vi "LauncherFeeder.vi"(3 "Target RPM F":dbl=770.0, 4 "Target RPM":dbl=3300.0) -> (0 "RPM F":dbl=3319.8279051826034, 1 "RPM L":dbl=3319.8279051826034)   [LabVIEW 2016]
doc: "This example shows how to move a motor connected to an encoder and a wheel, and then read information about the system from an encoder.\n\nThis is an example of how to use feedback (from the encoder) to create an open loop system. If some control method was used, for example using PID, a closed loop system could be created.\n\nThis example expects a USB cable connected from your development PC to the Type B USB Jack (next to the power input) on the roboRIO.\n\nThis example requires the Driver Station to be running with Teleoperated Enabled."
uses:
  <vilib>/Rock Robotics/WPI/Utilities/WPI_GetSetVariantRefNum.vi
  <vilib>/gmath/NI_Gmath.lvlib
panel:
  in  "Feeder Enabled":bool=TRUE
  out "DS Original F":dbl=0.6428571428571428
  in  "Lower Limit F":dbl=-50.0 format="%#_13g"
  in  "Upper Limit F":dbl=50.0 format="%#_13g"
  in  "Pos Drive Signal F":dbl=0.4
  in  "Neg Drive Signal F":dbl=0.05
  out "Error F":dbl=-19.827905182603445
  out "Encoder Alarm Status F":string="Encoder Moving"
  out "Encoder Direction F":string="Forward"
  in  "Lower Limit L":dbl=-50.0 format="%#_13g"
  in  "Upper Limit L":dbl=50.0 format="%#_13g"
  out "Error L":dbl=-19.827905182603445
  out "DS Original L":dbl=0.6428571428571428
  in  "Neg Drive Signal":dbl=0.6
  in  "Pos Drive Signal":dbl=1.0
  in  "MS to Wait":u32=10
  out "Loop Time (s)":dbl=0.010378 format="%_6f"
  out "Encoder Alarm Status L":string="Encoder Moving"
  out "Encoder Direction L":string="Forward"
  # "These can be set while running."
  # "Output information."
  # "Need to tune target RPM and drive signals"
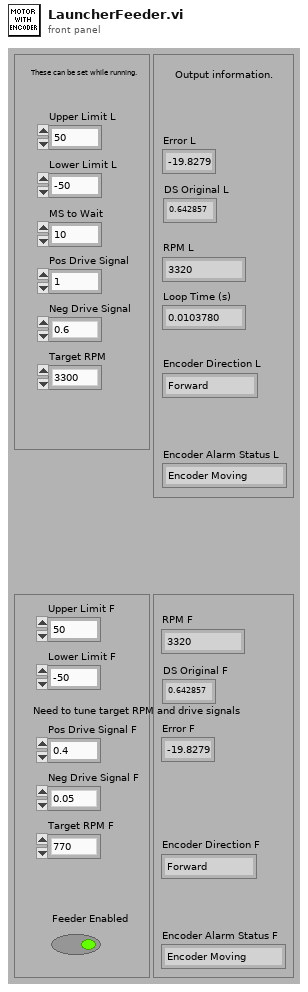
[diagram p1: front panel]
types:
  T1 = typedef "WPI_EncoderDevRef.ctl" = cluster{"DevStatus":errorcluster, "EncoderIndex":T2, "CounterIndex":T3, "DistancePerCount":dbl, "Decoding Type":T4}
  T2 = typedef "FPGA_EncoderIdx.ctl" = enum8{"Enc 0", "Enc 1", "Enc 2", "Enc 3", "Enc 4", "Enc 5", "Enc 6", "Enc 7", "Invalid"}
  T3 = typedef "FPGA_CounterCtrSystemIndex.ctl" = enum8{"Ctr 0", "Ctr 1", "Ctr 2", "Ctr 3", "Ctr 4", "Ctr 5", "Ctr 6", "Ctr 7", "Invalid"}
  T4 = typedef "WPI_EncoderType.ctl" = enum16{"1x", "2x", "4x"}
  T5 = typedef "WPI_MotorControlDeviceRef.ctl" = cluster{"DeviceStatus":errorcluster, "Type":T6, "PWM":cluster{"PWM Channel":T7, "DeadBand":T8}, "CAN":cluster{"Device Number":u8, "SetOutput VI Ref":variant, "GetOutput VI Ref":variant, "Enable VI Ref":variant, "Disable VI Ref":variant, "Data":variant}, "Invert":bool}
  T6 = typedef "WPI_MotorControlType.ctl" = enum16{"PWM", "CAN"}
  T7 = typedef "FPGA_DIOPWMChannel.ctl" = enum8{"PWM 0", "PWM 1", "PWM 2", "PWM 3", "PWM 4", "PWM 5", "PWM 6", "PWM 7", "PWM 8", "PWM 9", "PWM MXP 0", "PWM MXP 1", "PWM MXP 2", "PWM MXP 3", "PWM MXP 4", "PWM MXP 5", "PWM MXP 6", "PWM MXP 7", "PWM MXP 8", "PWM MXP 9", "Invalid"}
  T8 = typedef "WPI_PWMDeadband.ctl" = cluster{"Name":string, "maxPositivePwm":i32, "minPositivePwm":i32, "centerPwm":i32, "maxNegativePwm":i32, "minNegativePwm":i32, "angularRange":u16}
  T9 = typedef "WPI_JoystickDevRef.ctl" = cluster{"Device":T10}
  T10 = typedef "WPI_JoystickDeviceEnum.ctl" = enum16{"USB 0", "USB 1", "USB 2", "USB 3", "USB 4", "USB 5"}
  T11 = cluster{"Buttons[0]":bool, "Buttons[1]":bool, "Buttons[2]":bool, "Buttons[3]":bool, "Buttons[4]":bool, "Buttons[5]":bool, "Buttons[6]":bool, "Buttons[7]":bool, "Buttons[8]":bool}
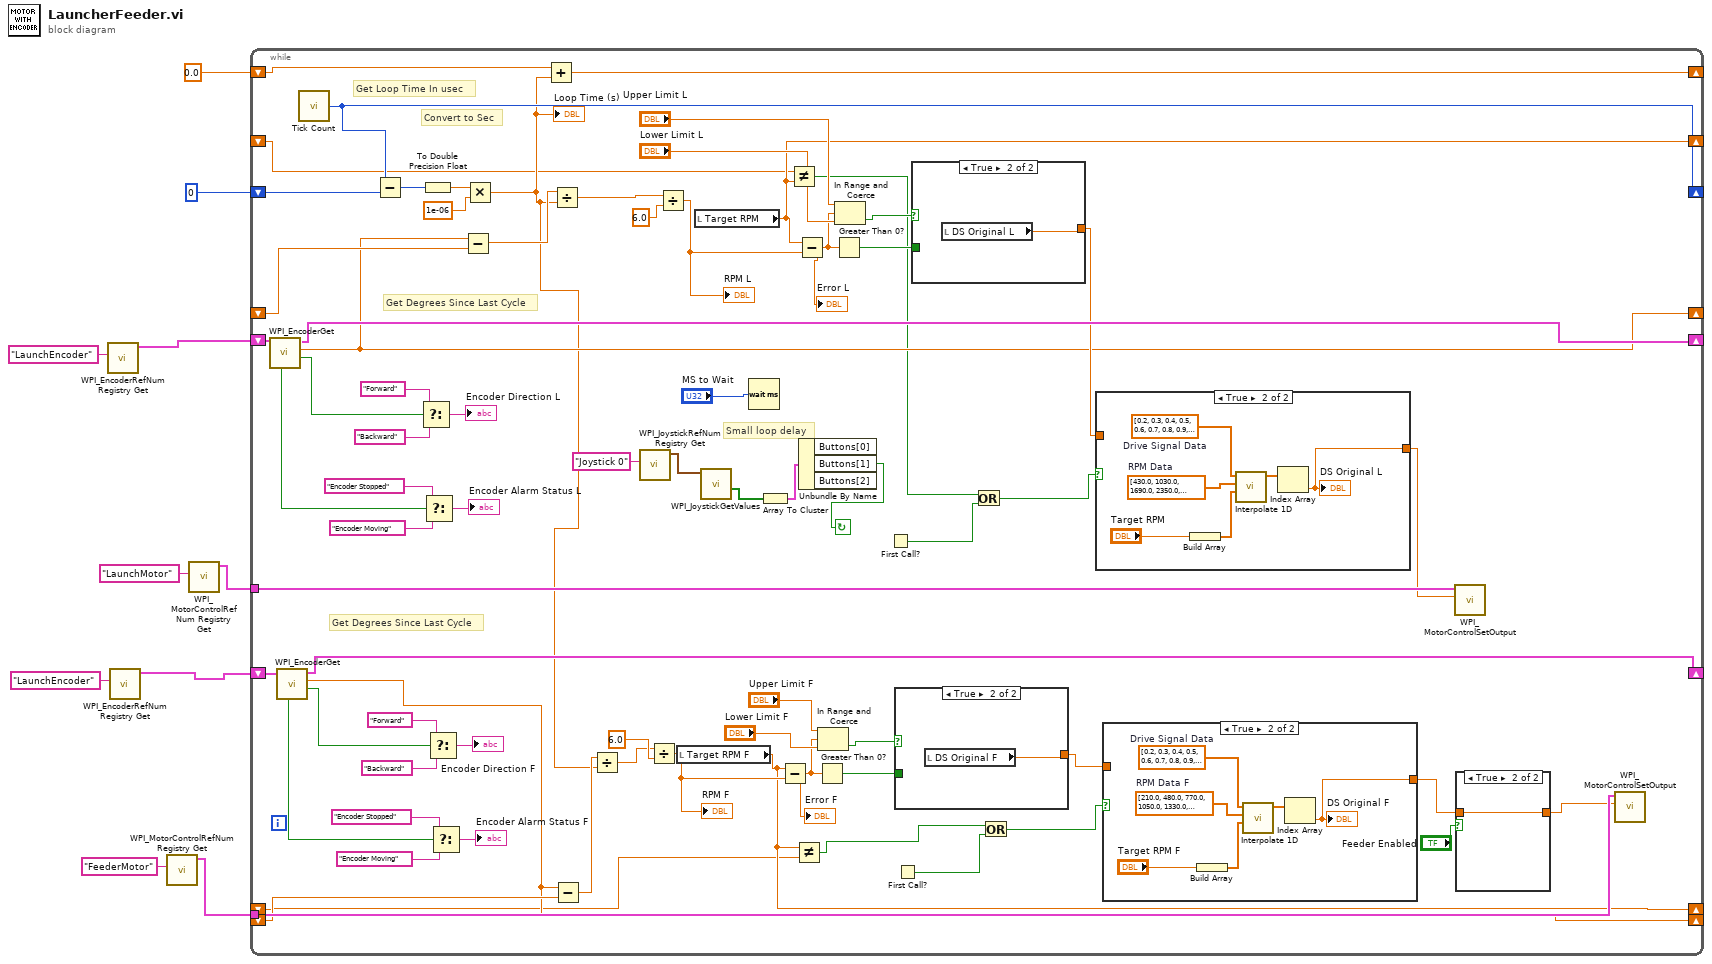
[diagram p0: block diagram]
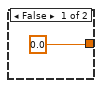
[diagram p2: hidden frame]
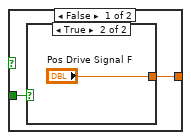
[diagram p4: hidden frame]
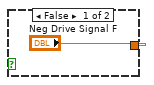
[diagram p5: hidden frame]
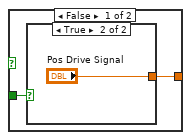
[diagram p7: hidden frame]
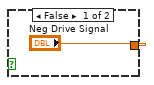
[diagram p8: hidden frame]
diagram:
  n1 = call <vilib>:"WPI_EncoderRefNum Registry Get.vi"("refnum name"="LaunchEncoder") -> ("EncoderDevRef"=w1:T1)  [unwired: 9 in, 1 out]
  n2 = call <vilib>:"WPI_EncoderRefNum Registry Get.vi"("refnum name"="LaunchEncoder") -> ("EncoderDevRef"=w2:T1)  [unwired: 9 in, 1 out]
  n3 = call <vilib>:"WPI_MotorControlRefNum Registry Get.vi"("refnum name"="FeederMotor") -> ("MotorControlDevRef"=w5:T5)  [unwired: 9 in, 1 out]
  n4 = call <vilib>:"WPI_MotorControlRefNum Registry Get.vi"("refnum name"="LaunchMotor") -> ("MotorControlDevRef"=w7:T5)  [unwired: 9 in, 1 out]
  n5 = while {
    shift-right: [w72] -> _
    shift-left: w1 -> [w75]
    tunnel: w7 -> [w76]
    shift-right: [w71] -> _
    shift-left: u32 0 ("Tick Count(uSec)") -> [w70]
    shift-right: [w51] -> _
    shift-left: _ -> [w69]
    shift-right: [w62] -> _
    shift-left: 0.0 ("Tick Count(uSec)") -> [w63]
    tunnel: w5 -> [w31]
    shift-right: [w29] -> _
    shift-left: w2 -> [w30]
    shift-right: [w23] -> _
    shift-left: _ -> [w27]
    shift-right: [w21] -> _
    shift-left: _ -> [w20]
    shift-right: [w18] -> _
    shift-left: _ -> [w17]
    stop <- w11 continue-if-true
    # "Get Degrees Since Last Cycle"
    # "Get Degrees Since Last Cycle"
    # "Convert to Sec"
    # "Get Loop Time In usec"
    # "Small loop delay"
    n6 = call <vilib>:"WPI_EncoderGet.vi"("EncoderDevRef"=w75) -> ("Direction"=w82:bool, "Distance"=w51:dbl, "EncoderDevRef"=w72:T1, "Stopped"=w81:bool)  [unwired: 1 in, 6 out]
    n7 = call <vilib>:"WPI_EncoderGet.vi"("EncoderDevRef"=w30) -> ("Direction"=w48:bool, "Distance"=w23:dbl, "EncoderDevRef"=w29:T1, "Stopped"=w47:bool)  [unwired: 1 in, 6 out]
    n8 = call "Tick Count"() -> ("Tick Count(uSec)"=w71:u32)
    n9 = Subtract(x=w71, y=w70) -> (x-y=w68:u32)
    n10 = Select(t="Forward", s=w82, f="Backward") -> (s? t:f=→"Encoder Direction L":string)
    n11 = To Double Precision Float(number=w68) -> (double precision float=w66:dbl)
    n12 = Select(t="Encoder Stopped", s=w81, f="Encoder Moving") -> (s? t:f=→"Encoder Alarm Status L":string)
    n13 = Select(t="Forward", s=w48, f="Backward") -> (s? t:f=→"Encoder Direction F":string)
    n14 = Select(t="Encoder Stopped", s=w47, f="Encoder Moving") -> (s? t:f=→"Encoder Alarm Status F":string)
    n15 = Subtract(x=w51, y=w69) -> (x-y=w65:dbl)
    n16 = Multiply(x=w66, y=1e-06) -> (x*y=w22:dbl)
    "Loop Time (s)" <- w22
    n17 = Add(x=w63, y=w22) -> (x+y=w62:dbl)
    n18 = Divide(x=w65, y=w22) -> (x/y=w64:dbl)
    n19 = Subtract(x=w23, y=w27) -> (x-y=w41:dbl)
    n20 = Divide(x=w41, y=w22) -> (x/y=w40:dbl)
    n21 = call <vilib>:"WPI_JoystickRefNum Registry Get.vi"("refnum name"="Joystick 0") -> ("JoystickDevRef"=w15:T9)  [unwired: 9 in, 1 out]
    n22 = Divide(x=w40, y=6.0) -> (x/y=w32:dbl)
    "RPM F" <- w32
    n23 = Divide(x=w64, y=6.0) -> (x/y=w61:dbl)
    "RPM L" <- w61
    n24 = local read "Target RPM F"() -> (w18:dbl)
    n25 = local read "Target RPM"() -> (w21:dbl)
    n26 = call <vilib>:"WPI_JoystickGetValues.vi"("JoystickDevRef"=w15) -> ("Buttons"=w13:bool[])  [unwired: 6 in, 4 out]
    n27 = Wait (ms)(milliseconds to wait="MS to Wait") -> ()  [unwired: 1 out]
    n28 = Array To Cluster(array=w13) -> (cluster=w12:T11)
    n29 = Subtract(x=w18, y=w32) -> (x-y=w35:dbl)
    "Error F" <- w35
    n30 = Not Equal?(x=w20, y=w21) -> (x != y?=w19:bool)
    n31 = Not Equal?(x=w18, y=w17) -> (x != y?=w16:bool)
    n32 = Subtract(x=w21, y=w61) -> (x-y=w56:dbl)
    "Error L" <- w56
    n33 = Unbundle By Name(w12) -> ("Buttons[1]"=w11:bool)  [unwired: 2 out]
    n34 = Greater Than 0?(x=w35) -> (x > 0?=w39:bool)
    n35 = In Range and Coerce(upper limit="Upper Limit F", x=w35, lower limit="Lower Limit F") -> (In Range?=w36:bool)  [unwired: 1 out]
    n36 = Greater Than 0?(x=w56) -> (x > 0?=w60:bool)
    n37 = In Range and Coerce(upper limit="Upper Limit L", x=w56, lower limit="Lower Limit L") -> (In Range?=w57:bool)  [unwired: 1 out]
    n38 = First Call?() -> (First Call?: T/F=w52:bool)
    n39 = First Call?() -> (First Call?: T/F=w33:bool)
    n40 = case shown="True" w36 {
      tunnel: w39 -> [w95 _]
      tunnel: [w94 w98] -> w28
      frame False {
        n41 = case shown="True" w95 {
          tunnel: ["Neg Drive Signal F" "Pos Drive Signal F"] -> w94
          frame False {
          }
          frame True {
          }
        }
      }
      frame True {
        n42 = local read "DS Original F"() -> (w98:dbl)
      }
    }
    n43 = case shown="True" w57 {
      tunnel: w60 -> [w107 _]
      tunnel: [w106 w110] -> w55
      frame False {
        n44 = case shown="True" w107 {
          tunnel: ["Neg Drive Signal" "Pos Drive Signal"] -> w106
          frame False {
          }
          frame True {
          }
        }
      }
      frame True {
        n45 = local read "DS Original L"() -> (w110:dbl)
      }
    }
    n46 = Or(x=w19, y=w52) -> (x .or. y?=w53:bool)
    n47 = Or(x=w16, y=w33) -> (x .or. y?=w34:bool)
    n48 = case shown="True" w53 {
      tunnel: [w99 w100] -> w54
      tunnel: w55 -> [w99 _]
      frame False {
      }
      frame True {
        w105 = dbl[] [430.0, 1030.0, 1690.0, 2350.0, 3000.0, 3700.0, 4400.0, 5000.0, 5550.0]  # RPM Data
        w104 = dbl[] [0.2, 0.3, 0.4, 0.5, 0.6, 0.7, 0.8, 0.9, 1.0]  # Drive Signal Data
        n49 = Build Array("Target RPM") -> (w102:dbl[])
        n50 = call <vilib>:"Interpolate 1D.vi"("xi"=w102, "X"=w105, "Y"=w104) -> ("yi"=w101:dbl[])  [unwired: 6 in, 2 out]
        n51 = Index Array(array=w101) -> (element=w100:dbl)  [unwired: 1 in]
        "DS Original L" <- w100
      }
    }
    n52 = case shown="True" w34 {
      tunnel: [w87 w88] -> w26
      tunnel: w28 -> [w87 _]
      frame False {
      }
      frame True {
        w93 = dbl[] [210.0, 480.0, 770.0, 1050.0, 1330.0, 1650.0, 1870.0, 2140.0, 2400.0]  # RPM Data F
        w92 = dbl[] [0.2, 0.3, 0.4, 0.5, 0.6, 0.7, 0.8, 0.9, 1.0]  # Drive Signal Data
        n53 = Build Array("Target RPM F") -> (w90:dbl[])
        n54 = call <vilib>:"Interpolate 1D.vi"("xi"=w90, "X"=w93, "Y"=w92) -> ("yi"=w89:dbl[])  [unwired: 6 in, 2 out]
        n55 = Index Array(array=w89) -> (element=w88:dbl)  [unwired: 1 in]
        "DS Original F" <- w88
      }
    }
    n56 = call <vilib>:"WPI_MotorControlSetOutput.vi"("Output"=w54, "MotorControlDevRef"=w76) -> ()  [unwired: 2 in, 8 out]
    n57 = case shown="True" "Feeder Enabled" {
      tunnel: [0.0 w86] -> w25
      tunnel: w26 -> [_ w86]
      frame False {
      }
      frame True {
      }
    }
    n58 = call <vilib>:"WPI_MotorControlSetOutput.vi"("Output"=w25, "MotorControlDevRef"=w31) -> ()  [unwired: 2 in, 8 out]
  }
